vi "Solve1.vi"(8 "Error In":errorcluster, 11 "reference in":refnum<class "2020_20.lvclass">) -> (0 "Error Out":errorcluster, 2 "Result":u64, 3 "reference in":refnum<class "2020_20.lvclass">)   [LabVIEW 2020, in "2020_20.lvclass"]
uses:
  2020_20.lvclass
  private/MatchState.ctl
  Image.ctl
  2020_20.lvclass/2020_20.ctl
panel:
  out "Images 2":T1
  out "Images":T1
  out "42":T1
  out "0":T1
  out "71":T1
  out "Array":T3(array[cluster])
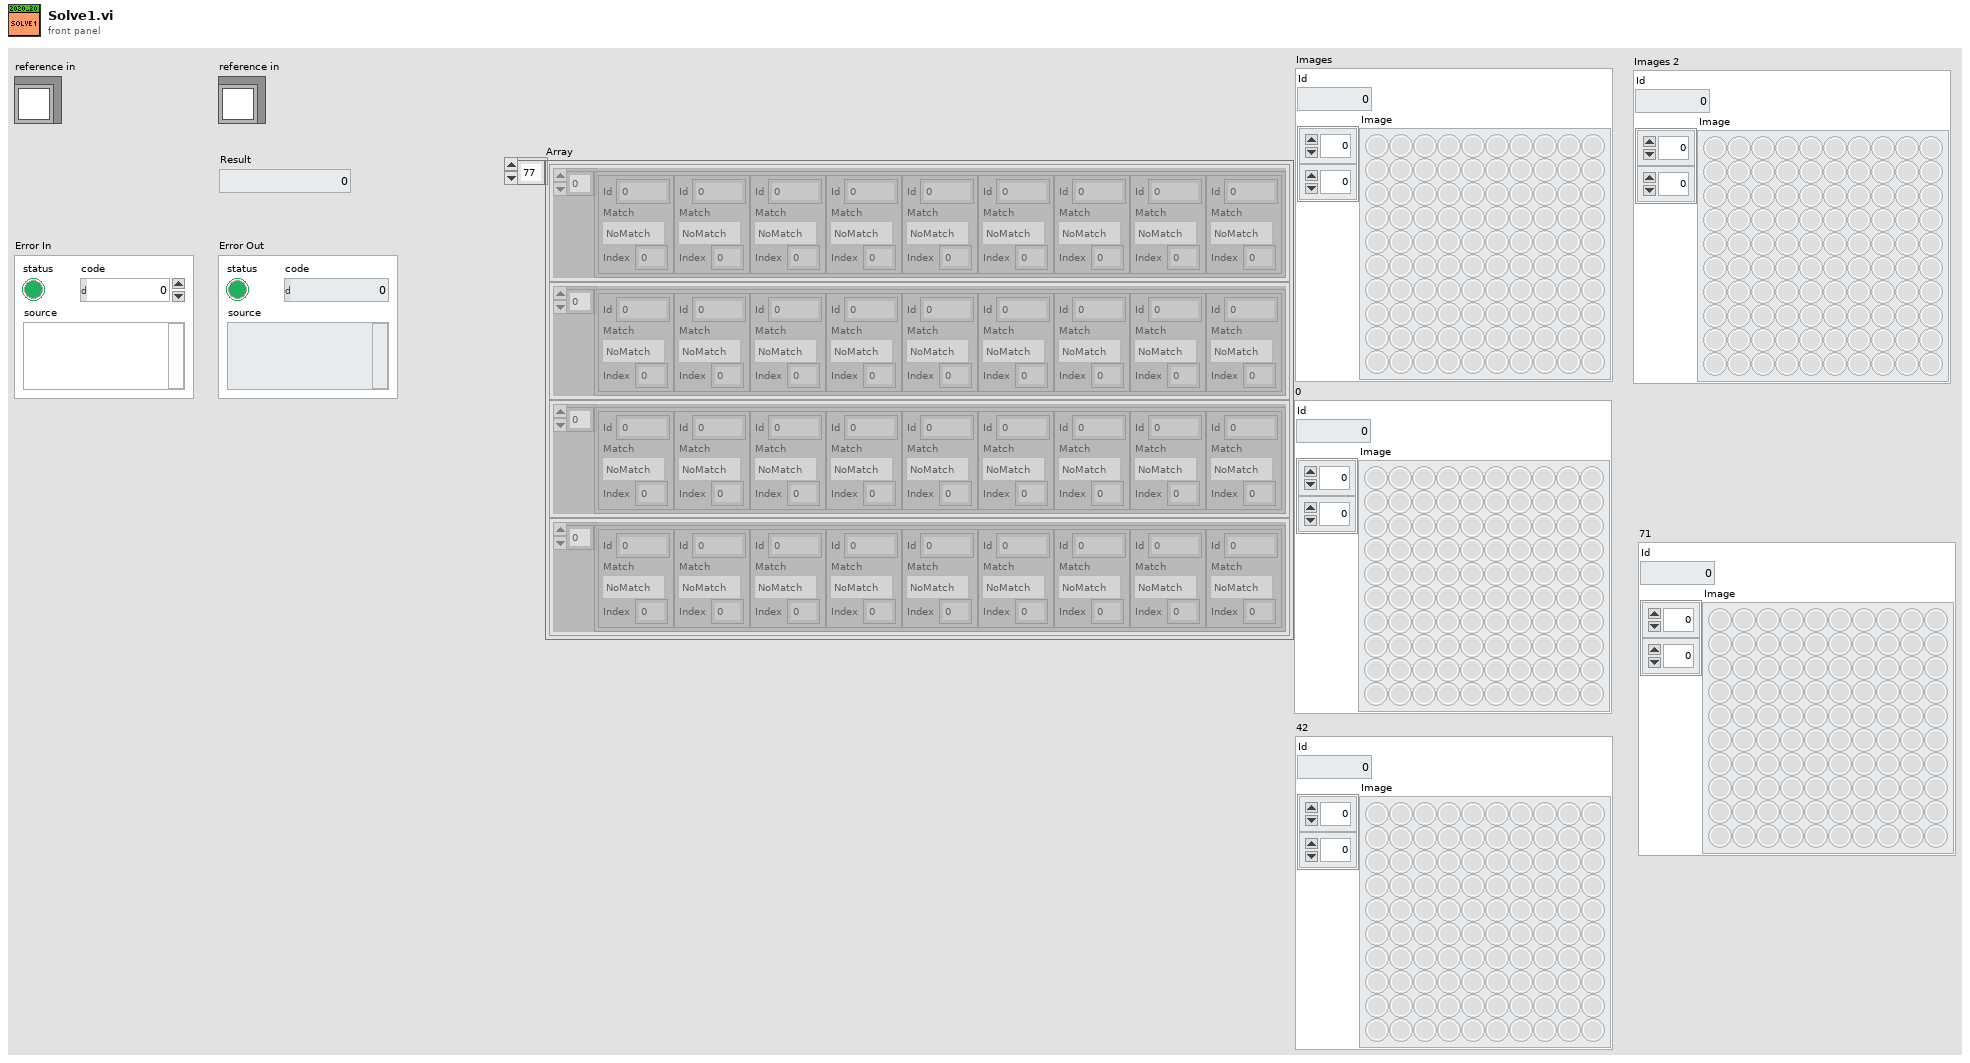
[diagram p1: front panel]
types:
  T1 = typedef "2020_20.lvclass/Image.ctl" = cluster{"Id":i32, "Image":bool[][]}
  T2 = typedef "2020_20.lvclass/MatchState.ctl" = enum16{"NoMatch", "Top", "Right", "Bottom", "Left"}
  T3 = cluster{cluster{"Id":i32, "Match":T2, "Index":i32}[]}[]
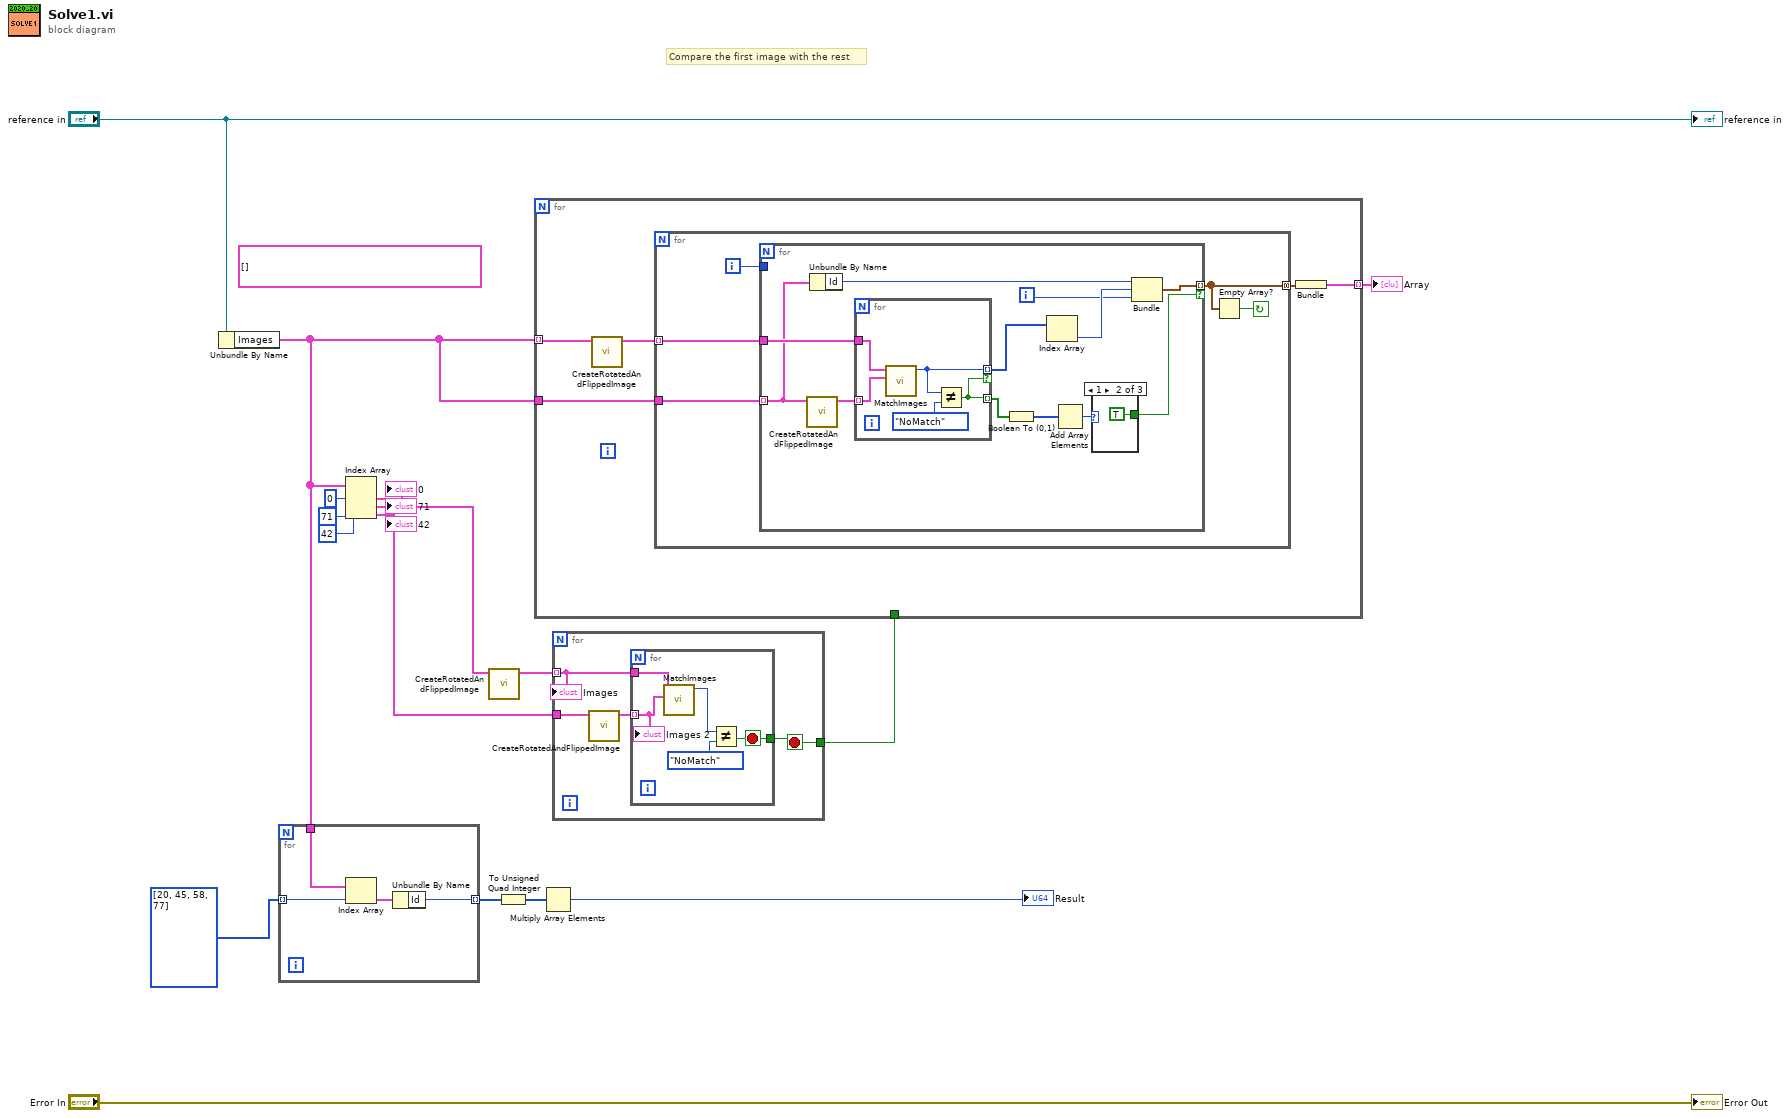
[diagram p0: block diagram]
diagram:
  (unwired) cluster{cluster{"Id":i32, "Direction":T2}[]}[] []
  # "Compare the first image with the rest"
  n1 = Unbundle By Name("reference in") -> ("Images"=w5:T1[])
  n2 = for {
    tunnel: w5 -> [w20]
    tunnel: i32[] [20, 45, 58, 77] ("index") -> [w19] mode=indexing
    tunnel: [w17] -> w3 mode=indexing
    n3 = Index Array(array=w20, index=w19) -> (element=w18:T1)
    n4 = Unbundle By Name(w18) -> ("Id"=w17:i32)
  }
  n5 = Index Array(array=w5, index #1=0 ("index"), index #2=71 ("index"), index #3=42 ("index")) -> (element #1=→"0":T1, element #2=w7:T1, element #3=w6:T1)
  "71" <- w7
  "42" <- w6
  n6 = call "CreateRotatedAndFlippedImage.vi"("ImageIn"=w7) -> ("RotatedAndFlipped"=w9:T1[])  [unwired: 9 in, 1 out]
  n7 = To Unsigned Quad Integer(1:w3) -> (0:w1:u64[])
  n8 = Multiply Array Elements(1:w1) -> (0:→"Result":u64)
  n9 = for {
    tunnel: w9 -> [w23] mode=indexing
    tunnel: w6 -> [w24]
    tunnel: [w21] -> w8
    stop <- w21 stop-if-true
    n10 = call "CreateRotatedAndFlippedImage.vi"("ImageIn"=w24) -> ("RotatedAndFlipped"=w22:T1[])  [unwired: 9 in, 1 out]
    n11 = for {
      tunnel: w23 -> [w29]
      tunnel: w22 -> [w28] mode=indexing
      tunnel: [w25] -> w21
      stop <- w25 stop-if-true
      n12 = call "MatchImages.vi"("Image2"=w28, "Image1"=w29) -> ("Match"=w26:T2)  [unwired: 9 in]
      n13 = Not Equal?(x=w26, y=MatchState."NoMatch") -> (x != y?=w25:bool)
      "Images 2" <- w28
    }
    "Images" <- w23
  }
  n14 = for {
    tunnel: w5 -> [w34] mode=indexing
    tunnel: w5 -> [w30]
    tunnel: [w31] -> w16 mode=indexing
    tunnel: w8 -> [_]
    n15 = call "CreateRotatedAndFlippedImage.vi"("ImageIn"=w34) -> ("RotatedAndFlipped"=w33:T1[])  [unwired: 9 in, 1 out]
    n16 = for {
      tunnel: w33 -> [w38] mode=indexing
      tunnel: w30 -> [w39]
      tunnel: [w37] -> w32 mode=concatenating
      i -> [w35]
      stop <- w36 continue-if-true
      n17 = for {
        tunnel: w39 -> [w49] mode=indexing
        tunnel: w38 -> [w50]
        tunnel: [w47] -> w37 mode=indexing if=w43
        tunnel: w35 -> [_]
        i -> [w40]
        n18 = call "CreateRotatedAndFlippedImage.vi"("ImageIn"=w49) -> ("RotatedAndFlipped"=w51:T1[])  [unwired: 9 in, 1 out]
        n19 = Unbundle By Name(w49) -> ("Id"=w48:i32)
        n20 = for {
          tunnel: w51 -> [w57] mode=indexing
          tunnel: w50 -> [w56]
          tunnel: [w55] -> w42 mode=indexing if=w53
          tunnel: [w53] -> w46 mode=indexing
          n21 = call "MatchImages.vi"("Image2"=w57, "Image1"=w56) -> ("Match"=w55:T2)  [unwired: 9 in]
          n22 = Not Equal?(x=w55, y=MatchState."NoMatch") -> (x != y?=w53:bool)
        }
        n23 = Boolean To (0,1)(Boolean=w46) -> (0, 1=w45:i16[])
        n24 = Index Array(array=w42) -> (element=w41:T2)  [unwired: 1 in]
        n25 = Add Array Elements(numeric array=w45) -> (sum=w44:i16)
        n26 = case shown="1" w44 {
          tunnel: [_ TRUE _] -> w43
          frame 0, Default {
          }
          frame 1 {
          }
          frame 2.. {
          }
        }
        n27 = Bundle("Id"=w48, "Match"=w41, w40) -> (w47:cluster{"Id":i32, "Match":T2, i32})  [unwired: 1 in]
      }
      n28 = Empty Array?(array=w37) -> (empty?=w36:bool)
    }
    n29 = Bundle(w32) -> (w31:cluster{cluster{"Id":i32, "Match":T2, i32}[]})  [unwired: 1 in]
  }
  "Array" <- w16
  "Error Out" <- "Error In"
  "reference in" <- "reference in"
